vi "Get Row Indexes Of Unread Errors.vi"(1 "Handled Errors (chronological order)":T1[](array[typedef])) -> (0 "Row Index Of Unread Errors":i32[](array[numeric]))   [LabVIEW 2016, in "Error Manager.lvlib"]
doc: "This VI returns the row indexes of rows that represent unread errors."
uses:
  Error Manager.lvlib
  Read-Unread Status (enum).ctl
  Handled Error (cluster).ctl
panel:
  # "Development\nControls or indicators that are useful for development or testing, but which are not outputs of the VI."
  # "Input\nInputs to the VI"
  # "Output\nOutputs of the VI"
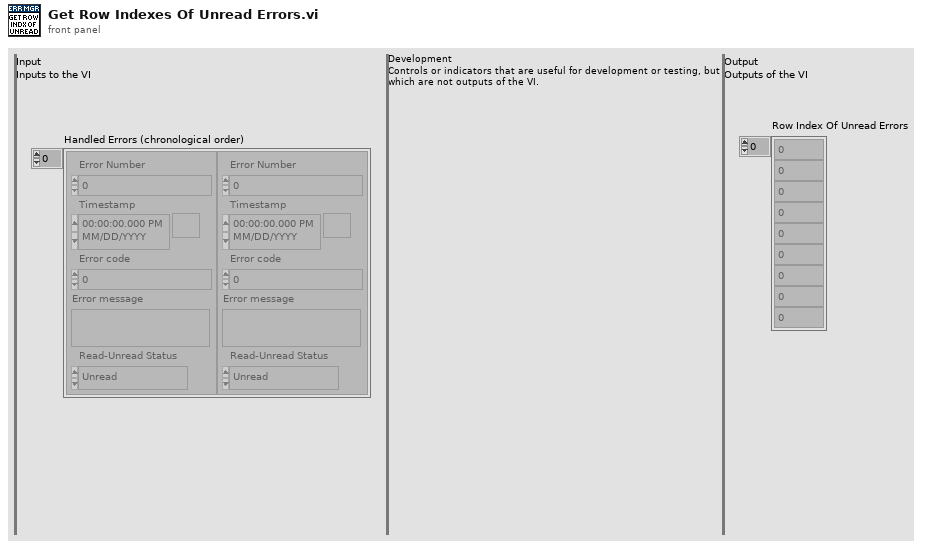
[diagram p1: front panel]
types:
  T1 = typedef "Error Manager.lvlib/Handled Error (cluster).ctl" = cluster{"Error Number":i32, "Timestamp":timestamp, "Error code":i32, "Error message":string, "Read-Unread Status":T2}
  T2 = typedef "Error Manager.lvlib/Read-Unread Status (enum).ctl" = enum16{"Unread", "Read"}
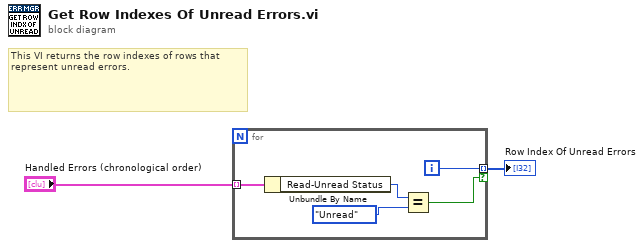
[diagram p0: block diagram]
diagram:
  # "This VI returns the row indexes of rows that represent unread errors."
  n1 = for {
    tunnel: "Handled Errors (chronological order)" -> [w6] mode=indexing
    tunnel: [w7] -> w1 mode=indexing if=w3
    i -> [w7]
    n2 = Unbundle By Name(w6) -> ("Read-Unread Status"=w5:T2)
    n3 = Equal?(x=w5, y=Read-Unread_Status_(enum)."Unread") -> (x = y?=w3:bool)
  }
  "Row Index Of Unread Errors" <- w1
